vi "WRYield.vi"(0 "Pass in":dbl, 1 "RW":enum16{"Read", "Write"}(ring), 5 "Fail in":dbl, 7 "Error in":dbl, 9 "Yield in":dbl, 11 "error in (no error)":errorcluster caption="错误输入（无错误）") -> (4 "Pass out":dbl, 6 "Fail out":dbl, 8 "Error out":dbl, 10 "Yield out":dbl, 15 "error out":errorcluster caption="错误输出")   [LabVIEW 2024]
uses:
  <vilib>/Utility/config.llb/Read Key (Double).vi
  <vilib>/Utility/config.llb/Write Key (Double).vi
  <vilib>/Utility/config.llb/NI_LVConfig.lvlib
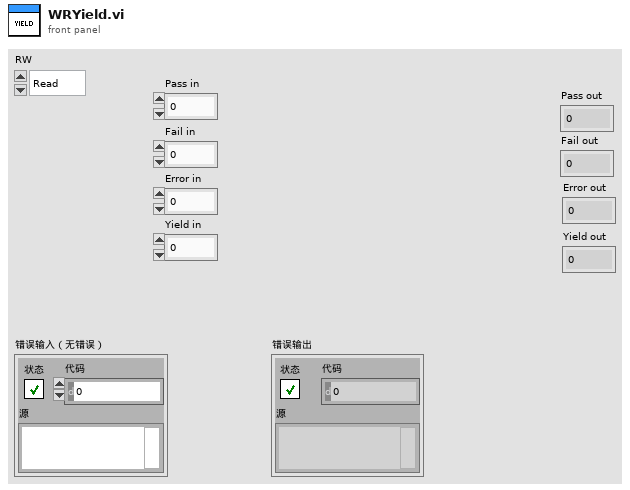
[diagram p1: front panel]
types:
  T1 = typedef "NI_LVConfig.lvlib/Config Data RefNum.ctl" = refnum<k1>
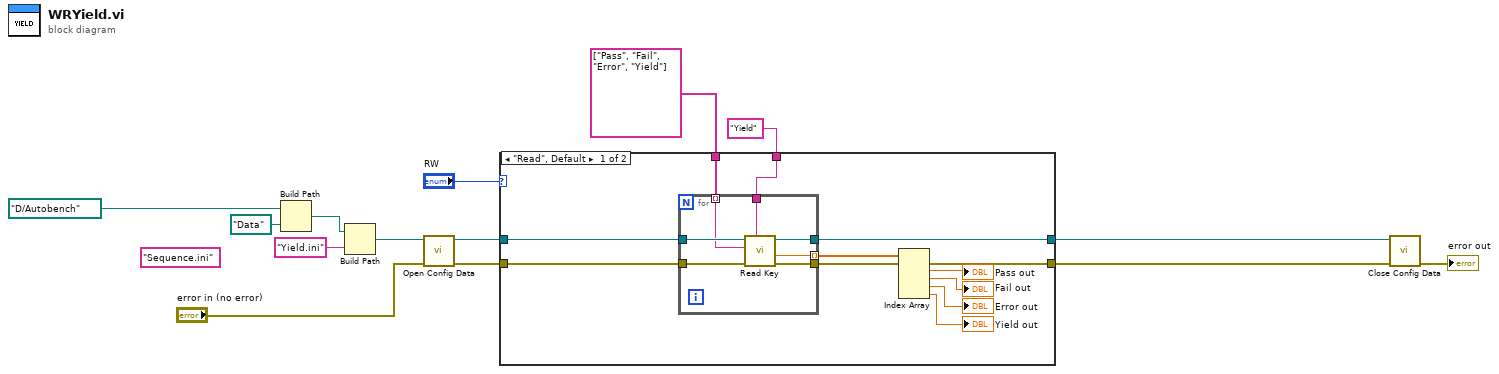
[diagram p0: block diagram]
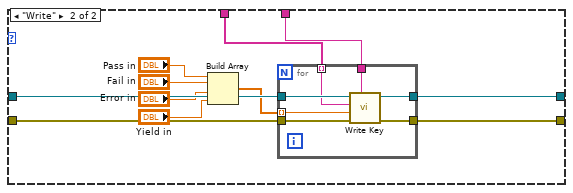
[diagram p2: hidden frame]
diagram:
  (unwired) "Sequence.ini" ("name or relative path")
  n1 = Build Path(base path=path "D:/Autobench", name or relative path=path "Data") -> (appended path=w12:path)
  n2 = Build Path(base path=w12, name or relative path="Yield.ini") -> (appended path=w11:path)
  n3 = call <vilib>:"Open Config Data.vi"("error in (no error)"="error in (no error)", "configuration file path"=w11) -> ("error out"=w9:errorcluster, "refnum"=w8:T1)  [unwired: 7 in, 1 out]
  n4 = case shown="\"Read\", Default" "RW" {
    tunnel: w9 -> [w24 w43]
    tunnel: w8 -> [w25 w42]
    tunnel: [w22 w41] -> w7
    tunnel: [w23 w40] -> w6
    tunnel: "Yield" ("section") -> [w21 w39]
    tunnel: string[] ["Pass", "Fail", "Error", "Yield"] -> [w20 w38]
    frame "Read", Default {
      n5 = for {
        tunnel: w21 -> [w28]
        tunnel: w25 -> [w32]
        tunnel: [w30] -> w23
        tunnel: w24 -> [w31]
        tunnel: [w29] -> w22
        tunnel: w20 -> [w27] mode=indexing
        tunnel: [w26] -> w19 mode=indexing
        n6 = call-poly <vilib>:"Read Key.vi"("section"=w28, "error in (no error)"=w31, "key"=w27, "refnum"=w32) -> ("error out"=w29:errorcluster, "value"=w26:dbl, "refnum out"=w30:T1)  [unwired: 4 in, 1 out]
      }
      n7 = Index Array(array=w19) -> (element #1=→"Pass out":dbl, element #2=→"Fail out":dbl, element #3=→"Error out":dbl, element #4=→"Yield out":dbl)  [unwired: 4 in]
    }
    frame "Write" {
      n8 = Build Array("Pass in", "Fail in", "Error in", "Yield in") -> (w36:dbl[])
      n9 = for {
        tunnel: w39 -> [w46]
        tunnel: w42 -> [w49]
        tunnel: [w47] -> w40
        tunnel: w43 -> [w50]
        tunnel: [w48] -> w41
        tunnel: w38 -> [w45] mode=indexing
        tunnel: w36 -> [w44] mode=indexing
        n10 = call-poly <vilib>:"Write Key.vi"("section"=w46, "error in (no error)"=w50, "value"=w44, "key"=w45, "refnum"=w49) -> ("error out"=w48:errorcluster, "refnum out"=w47:T1)  [unwired: 4 in, 1 out]
      }
    }
  }
  n11 = call <vilib>:"Close Config Data.vi"("error in (no error)"=w7, "refnum"=w6) -> ("error out"=→"error out":errorcluster)  [unwired: 8 in, 1 out]
